vi "Vision Processing.vi"(4 "error in (no error)":errorcluster) -> ()   [LabVIEW 2012]
doc: "This VI runs in parallel to other tasks. It gets images from the camera, processes them for color or shape and use that information to affect robot behavior."
uses:
  Robot Global Data.vi
panel:
  out "2D Picture":picture
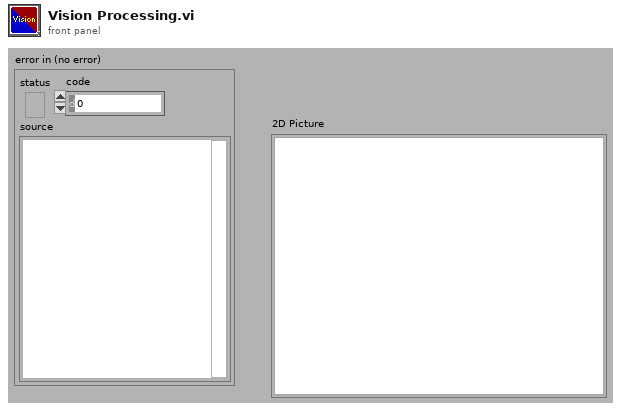
[diagram p1: front panel]
types:
  T1 = typedef "Image Type" = u32
  T2 = typedef "WPI_CameraDevRef.ctl" = cluster{"Camera Address":string, "CameraStatus":errorcluster, "Acquire Image Notifier":refnum<notifier>}
  T3 = typedef "IMAQ Image.ctl" = refnum<image>
  T4 = typedef "WPI_CameraImageSize.ctl" = enum16{"640x480", "320x240", "160x120"}
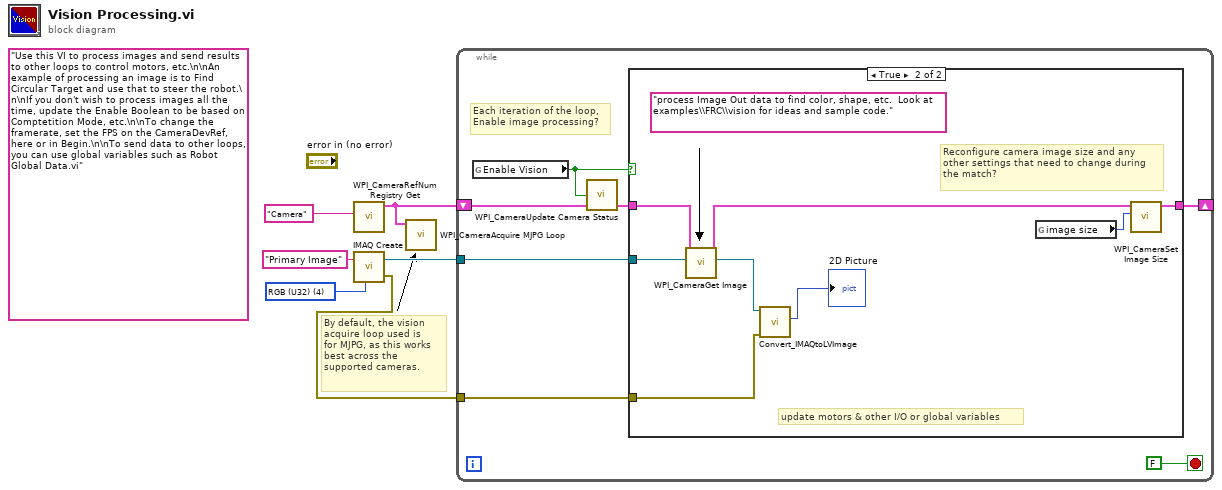
[diagram p0: block diagram]
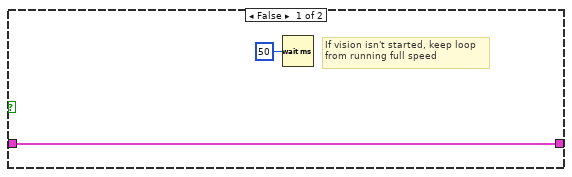
[diagram p2: hidden frame]
diagram:
  (unwired) "Use this VI to process images and send results to other loops to control motors, etc.\n\nAn example of processing an image is to Find Circular Target and use that to steer the robot.\n\nIf you don't wish to process images all the time, update the Enable Boolean to be based on Comptetition Mode, etc.\n\nTo change the framerate, set the FPS on the CameraDevRef, here or in Begin.\n\nTo send data to other loops, you can use global variables such as Robot Global Data.vi"
  w6 = T1 4 items=["Grayscale (U8)", "Grayscale (I16)", "Grayscale (SGL)", "Complex (CSG)", "RGB (U32)", "HSL (U32)", "RGB (U64)"] ("Image Type")
  # "By default, the vision\nacquire loop used is\nfor MJPG, as this works\nbest across the\nsupported cameras."
  n1 = call <vilib>:"WPI_CameraRefNum Registry Get.vi"("refnum name"="Camera") -> ("CameraDevRef"=w2:T2)  [unwired: 1 in, 9 out]
  n2 = call "IMAQ Create"("Image Name"="Primary Image", "Image Type"=w6) -> ("New Image"=w4:T3, "error out"=w1:errorcluster)  [unwired: 2 in, 1 out]
  n3 = call <vilib>:"WPI_CameraAcquire MJPG Loop.vi"("CameraDevRef"=w2) -> ()  [unwired: 11 in]
  n4 = while {
    shift-right: [w12] -> _
    shift-left: w2 -> [w10]
    tunnel: w4 -> [w11]
    tunnel: w1 -> [w7]
    stop <- FALSE stop-if-true
    # "Each iteration of the loop,\nEnable image processing?"
    n5 = global read "Robot Global Data.vi" "Enable Vision"() -> (w8:bool)
    n6 = call <vilib>:"WPI_CameraUpdate Camera Status.vi"("CameraDevRef In"=w10, "Enable Vision"=w8) -> ("CameraDevRef Out"=w9:T2)  [unwired: 3 in]
    n7 = case shown="True" w8 {
      tunnel: w11 -> [_ w22]
      tunnel: [w15 w23] -> w12
      tunnel: w9 -> [w15 w20]
      tunnel: w7 -> [_ w16]
      frame False {
        # "If vision isn't started, keep loop\nfrom running full speed"
        n8 = Wait (ms)(milliseconds to wait=u32 50) -> ()  [unwired: 1 out]
      }
      frame True {
        (unwired) "process Image Out data to find color, shape, etc.  Look at examples\\FRC\\vision for ideas and sample code."
        # "update motors & other I/O or global variables"
        # "Reconfigure camera image size and any\nother settings that need to change during\nthe match?"
        n9 = call <vilib>:"WPI_CameraGet Image.vi"("Image"=w22, "CameraDevRef"=w20) -> ("Image Out"=w17:T3, "CameraDevRef Out"=w19:T2)  [unwired: 1 in, 7 out]
        n10 = call "Convert_IMAQtoLVImage.vi"("Error In"=w16, "IMAQImage In (RGB 32)"=w17) -> ("Image 2D"=→"2D Picture":picture)  [unwired: 6 in, 3 out]
        n11 = global read "Robot Global Data.vi" "image size"() -> (w21:T4)
        n12 = call <vilib>:"WPI_CameraSet Image Size.vi"("Image Size"=w21, "CameraDevRef"=w19) -> ("CameraDevRef Out"=w23:T2)  [unwired: 1 in, 8 out]
      }
    }
  }
